vi "CCD Image Information.vi"(8 "Error In":errorcluster, 10 "CCD Image settings In":T1={"Image Size"={"Height"=0, "Width"=0}, "exposure range"={"min"=0.0, "max"=0.0, "intervall"=0.0}, "exposure time"=0.0, "Pixel Clock"=0, "Bits/Pixel"=8}, 11 "mode (R)":T2=enum."read") -> (0 "Error out":errorcluster, 2 "CCD Image settings Out":T1={"Image Size"={"Height"=0, "Width"=0}, "exposure range"={"min"=0.0, "max"=0.0, "intervall"=0.0}, "exposure time"=0.0, "Pixel Clock"=0, "Bits/Pixel"=8})   [LabVIEW 2011]
doc: "Functional Global Variable for the algorithm settings. The used method as well as the max. Iteration steps and the tolerance can be given. In addition, the algorithm can be told to use boundaries (if possible)."
uses:
  controls/FGV_Action.ctl
  controls/CCD Image Information.ctl
panel:
  # "Input"
  # "Output"
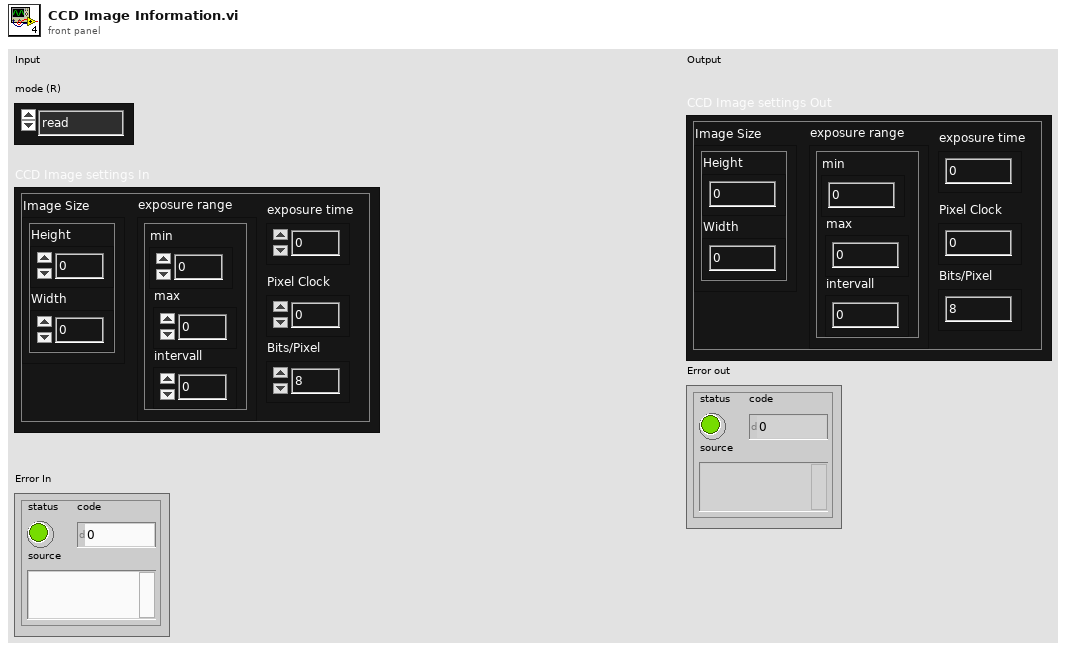
[diagram p1: front panel]
types:
  T1 = typedef "CCD Image Information.ctl" = cluster{"Image Size":cluster{"Height":i32, "Width":i32}, "exposure range":cluster{"min":dbl, "max":dbl, "intervall":dbl}, "exposure time":dbl, "Pixel Clock":i32, "Bits/Pixel":i32}
  T2 = typedef "FGV_Action.ctl" = enum16{"set to default", "read", "write"}
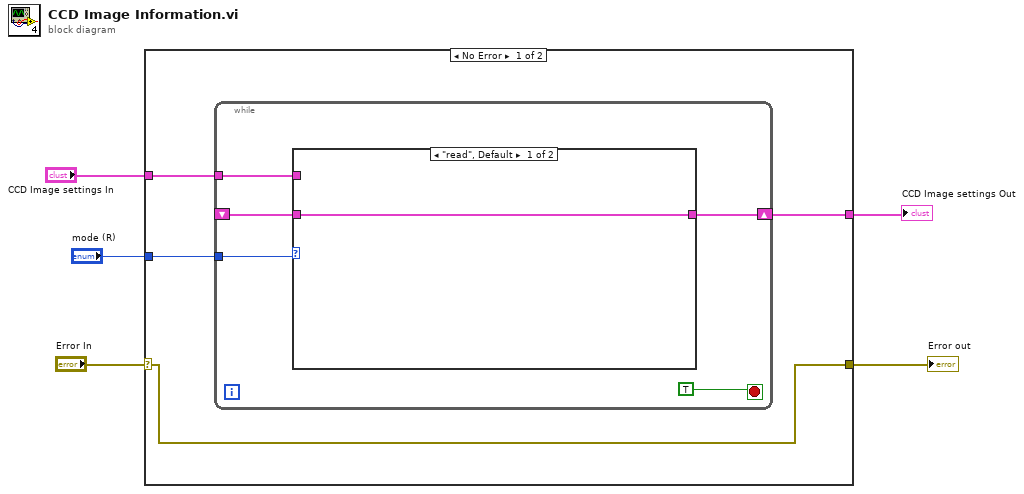
[diagram p0: block diagram]
diagram:
  n1 = case shown="No Error" "Error In" {
    selector: "Error In" -> [w6 w18]
    tunnel: "mode (R)" -> [w9 _]
    tunnel: [w6 w18] -> w3
    tunnel: "CCD Image settings In" -> [w8 w17]
    tunnel: [w7 w17] -> w1
    frame No Error {
      n2 = while {
        tunnel: w9 -> [w13]
        tunnel: w8 -> [w12]
        shift-right: [w10] -> w7
        shift-left: _ -> [w11]
        stop <- TRUE stop-if-true
        n3 = case shown="\"read\", Default" w13 {
          tunnel: w12 -> [_ w16]
          tunnel: w11 -> [w15 _]
          tunnel: [w15 w16] -> w10
          frame "read", Default {
          }
          frame "write" {
          }
        }
      }
    }
    frame Error {
    }
  }
  "Error out" <- w3
  "CCD Image settings Out" <- w1
